vi "meth.CallModuleStatic.vi"(0 "GLue in":refnum<class "class.GLue.lvclass">, 11 "error in":errorcluster) -> (4 "GLue out":refnum<class "class.GLue.lvclass">, 13 "Data Out":variant, 15 "error out":errorcluster)   [LabVIEW 2014, in "GLue.lvlib" / "class.GLue.lvclass"]
uses:
  class.GLue.lvclass
  class.GLue.lvclass/class.GLue.ctl
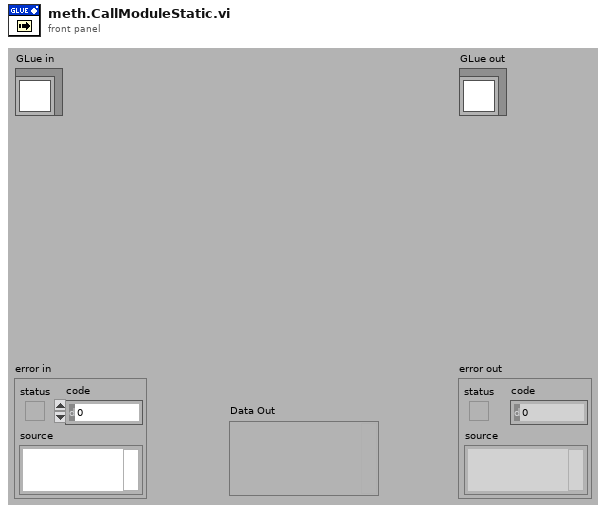
[diagram p1: front panel]
types:
  T1 = typedef "GLue.lvlib/class.GLue.lvclass/typedef.LVCallData.ctl" = cluster{"Command":string, "Data":variant}
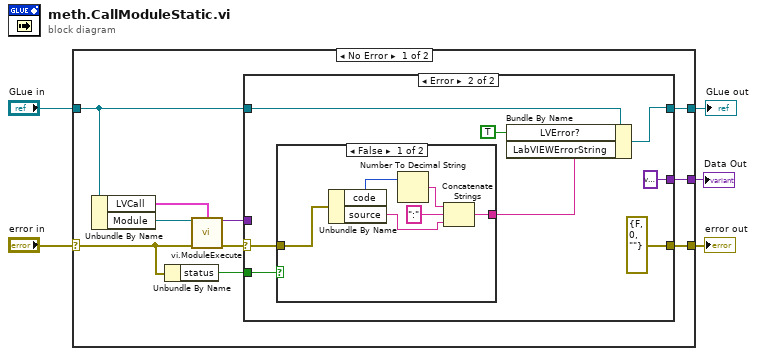
[diagram p0: block diagram]
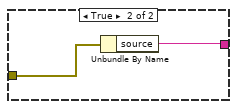
[diagram p3: hidden frame]
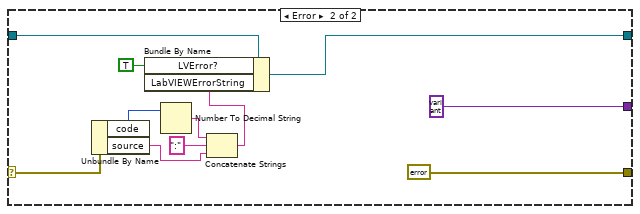
[diagram p4: hidden frame]
diagram:
  n1 = case shown="No Error" "error in" {
    selector: "error in" -> [w7 w36]
    tunnel: [w13 errorcluster {"status"=FALSE, "code"=0, "source"=""} ("error IO")] -> w4
    tunnel: [w15 w37] -> w2
    tunnel: "GLue in" -> [w9 w38]
    tunnel: [w14 variant ("Data Out")] -> w1
    frame No Error {
      n2 = Unbundle By Name(w9) -> ("LVCall"=w8:T1, "Module"=w6:refnum<vi>)
      n3 = Unbundle By Name(w7) -> ("status"=w10:bool)
      n4 = call "vi.ModuleExecute.vi"("Module"=w6, "LVCall"=w8, "error in"=w7) -> ("Return Data"=w11:variant, "error out"=w12:errorcluster)  [unwired: 11 in]
      n5 = case shown="Error" w12 {
        selector: w12 -> [w16 w21]
        tunnel: w9 -> [w18 w26]
        tunnel: [w18 w25] -> w15
        tunnel: [w17 variant ("Data Out")] -> w14
        tunnel: w11 -> [w17 _]
        tunnel: [w16 errorcluster {"status"=FALSE, "code"=0, "source"=""} ("error IO")] -> w13
        tunnel: w10 -> [_ w19]
        frame No Error {
        }
        frame Error {
          n6 = case shown="False" w19 {
            tunnel: w21 -> [w32 w34]
            tunnel: [w27 w33] -> w20
            frame False {
              n7 = Unbundle By Name(w32) -> ("code"=w31:i32, "source"=w28:string)
              n8 = Number To Decimal String(number=w31) -> (decimal integer string=w30:string)  [unwired: 1 in]
              n9 = Concatenate Strings(w30, ":" ("string"), w28) -> (w27:string)
            }
            frame True {
              n10 = Unbundle By Name(w34) -> ("source"=w33:string)
            }
          }
          n11 = Bundle By Name(cluster=w26, "LVError?"=TRUE, "LabVIEWErrorString"=w20) -> (w25:refnum<class "class.GLue.lvclass">)
        }
      }
    }
    frame Error {
      n12 = Unbundle By Name(w36) -> ("code"=w43:i32, "source"=w40:string)
      n13 = Number To Decimal String(number=w43) -> (decimal integer string=w42:string)  [unwired: 1 in]
      n14 = Concatenate Strings(w42, ":" ("string"), w40) -> (w39:string)
      n15 = Bundle By Name(cluster=w38, "LVError?"=TRUE, "LabVIEWErrorString"=w39) -> (w37:refnum<class "class.GLue.lvclass">)
    }
  }
  "error out" <- w4
  "GLue out" <- w2
  "Data Out" <- w1
